vi "ini interface.vi"(0 "dataserver":string, 5 "Serial Port":refnum<visa-resource-name>="COM1", 7 "Stamp Model":string, 9 "dataserver list":string, 11 "Local Daq Config":T1={"Sample rate (Hz)"=1.0, "Over sample factor"=1.0, "Terminal Configuration"=enum."Single Ended", "Device"=0, "Max Voltage"=0} {"Max Voltage" items=["1", "1", "2", "2", "4", "5", "10", "20"]; "Device" items=["Dev1"]; "Over sample factor" min=1.0 max=250.0 step=1.0; "Sample rate (Hz)" min=1.0 max=10000.0 step=1.0}, 12 "direction":T2, 13 "ini interface":T3=enum."dataserver") -> (4 "dataserver out":string, 6 "Serial Port out":refnum<visa-resource-name>="COM1", 8 "Stamp Model":string, 10 "dataserver list out":string, 15 "Local Daq Config out":T1={"Sample rate (Hz)"=1.0, "Over sample factor"=1.0, "Terminal Configuration"=enum."Single Ended", "Device"=0, "Max Voltage"=0} {"Max Voltage" items=["1", "1", "2", "2", "4", "5", "10", "20"]; "Device" items=["Dev1"]; "Over sample factor" min=1.0 max=250.0 step=1.0; "Sample rate (Hz)" min=1.0 max=10000.0 step=1.0})   [LabVIEW 2015]
uses:
  <vilib>/Utility/config.llb/NI_LVConfig.lvlib
  Calibration and Function folders.ctl
  <vilib>/Utility/config.llb/Read Key (String).vi
  <vilib>/Utility/config.llb/Write Key (String).vi
  ini interface.ctl
  read-write.ctl
  Distributed Daq/Local Daq Config.ctl
panel:
  out "Ini file path":path
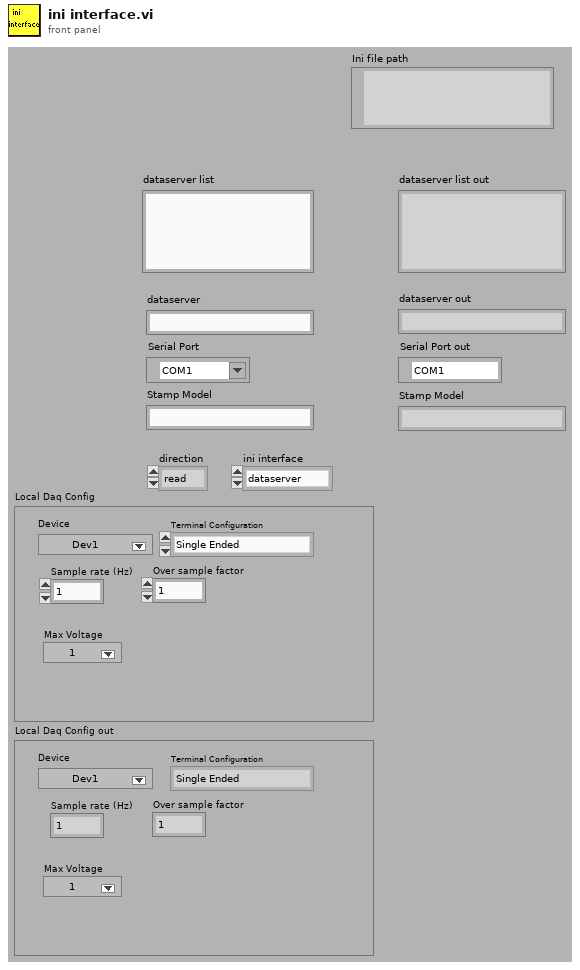
[diagram p1: front panel]
types:
  T1 = typedef "Local Daq Config.ctl" = cluster{"Sample rate (Hz)":dbl, "Over sample factor":dbl, "Terminal Configuration":enum16{"Single Ended", "Differential"}, "Device":u16, "Max Voltage":u16}
  T2 = typedef "read-write.ctl" = enum16{"read", "write"}
  T3 = typedef "ini interface.ctl" = enum16{"dataserver list", "dataserver", "com port", "stamp model", "Local Daq"}
  T4 = typedef "Calibration and Function folders.ctl" = enum16{"Sensors", "Functions", "Config File", "PublicAppFolder", "New ini File", "Set Config File", "Delete ini File"}
  T5 = typedef "NI_LVConfig.lvlib/Config Data RefNum.ctl" = refnum<k1>
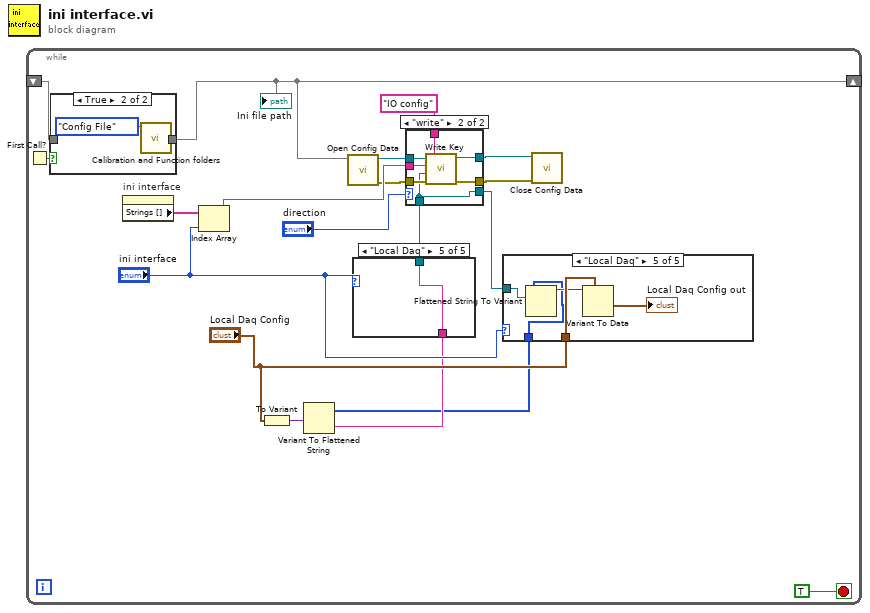
[diagram p0: block diagram]
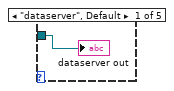
[diagram p2: hidden frame]
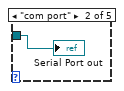
[diagram p3: hidden frame]
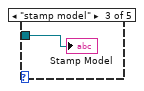
[diagram p4: hidden frame]
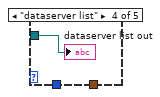
[diagram p5: hidden frame]
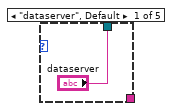
[diagram p6: hidden frame]
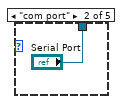
[diagram p7: hidden frame]
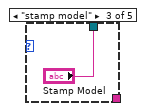
[diagram p8: hidden frame]
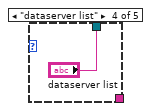
[diagram p9: hidden frame]
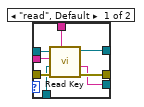
[diagram p10: hidden frame]
diagram:
  n1 = while {
    shift-right: [w11] -> _
    shift-left: _ -> [w17]
    stop <- TRUE stop-if-true
    n2 = First Call?() -> (First Call?: T/F=w18:bool)
    n3 = case shown="True" w18 {
      tunnel: [w49 w50] -> w11
      tunnel: w17 -> [w49 _]
      frame False {
      }
      frame True {
        n4 = call "Calibration and Function folders.vi"(11:Calibration_and_Function_folders."Config File" ("Folder")) -> (7:w50)  [unwired: 8 in, 2 out]
      }
    }
    "Ini file path" <- w11
    n5 = property on="ini interface" class="Enum (strict)"() -> ("Strings []"=w16:string[])  [unwired: 2 in, 2 out]
    n6 = Index Array(array=w16, index="ini interface") -> (element=w15:string)
    n7 = To Variant(anything="Local Daq Config") -> (Variant=w4:variant)
    n8 = Variant To Flattened String(Variant=w4) -> (data string=w2:string, 1:w1:i16[])
    n9 = call <vilib>:"Open Config Data.vi"("configuration file path"=w11) -> ("error out"=w12:errorcluster, "refnum"=w10:T5)  [unwired: 8 in, 1 out]
    n10 = case shown="\"Local Daq\"" "ini interface" {
      tunnel: ["dataserver" "Serial Port" "Stamp Model" "dataserver list" w33] -> w7
      tunnel: w2 -> [_ _ _ _ w33]
      frame "dataserver", Default {
      }
      frame "com port" {
      }
      frame "stamp model" {
      }
      frame "dataserver list" {
      }
      frame "Local Daq" {
      }
    }
    n11 = case shown="\"write\"" "direction" {
      tunnel: w15 -> [w41 w46]
      tunnel: "IO config" ("section") -> [w40 w43]
      tunnel: [w39 w48] -> w13
      tunnel: w12 -> [w38 w47]
      tunnel: w10 -> [w37 w45]
      tunnel: [w36 w44] -> w9
      tunnel: w7 -> [w34 w42]
      tunnel: [w35 w42] -> w5
      frame "read", Default {
        n12 = call-poly <vilib>:"Read Key.vi"("section"=w40, "error in (no error)"=w38, "default value"=w34, "key"=w41, "refnum"=w37) -> ("error out"=w39:errorcluster, "value"=w35:string, "refnum out"=w36:T5)  [unwired: 3 in, 1 out]
      }
      frame "write" {
        n13 = call-poly <vilib>:"Write Key.vi"("section"=w43, "error in (no error)"=w47, "value"=w42, "key"=w46, "refnum"=w45) -> ("error out"=w48:errorcluster, "refnum out"=w44:T5)  [unwired: 4 in, 1 out]
      }
    }
    n14 = case shown="\"Local Daq\"" "ini interface" {
      tunnel: w5 -> [w20 w21 w22 w23 w26]
      tunnel: "Local Daq Config" -> [_ _ _ _ w28]
      tunnel: w1 -> [_ _ _ _ w24]
      frame "dataserver", Default {
        "dataserver out" <- w20
      }
      frame "com port" {
        "Serial Port out" <- w21
      }
      frame "stamp model" {
        "Stamp Model" <- w22
      }
      frame "dataserver list" {
        "dataserver list out" <- w23
      }
      frame "Local Daq" {
        n15 = Flattened String To Variant(6:w26, 7:w24) -> (3:w25:variant)  [unwired: 1 in, 1 out]
        n16 = Variant To Data(type=w28, Variant=w25) -> (data=→"Local Daq Config out":T1)  [unwired: 1 in, 1 out]
      }
    }
    n17 = call <vilib>:"Close Config Data.vi"("error in (no error)"=w13, "refnum"=w9) -> ()  [unwired: 8 in, 2 out]
  }
